vi "SyntaxToken.vi"(8 "error in":errorcluster, 9 "Error Index In":i32, 10 "Funcion Analizada":string, 11 "Parsed Expression In":T1) -> (0 "error out":errorcluster, 1 "Error Index Out":i32, 2 "Token":string[](array[string]), 3 "Parsed Expression Out":T1)   [LabVIEW 2014, in "MathLoop.lvlib"]
uses:
  MathLoop.lvlib
  TypeDefs/ParsedExpression.ctl
  TypeDefs/typeMed.ctl
  <vilib>/regexp/Match Regular Expression.xnode
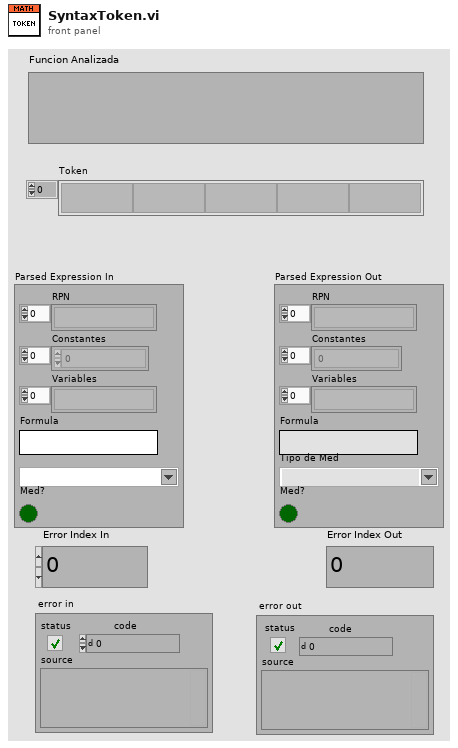
[diagram p1: front panel]
types:
  T1 = typedef "MathLoop.lvlib/ParsedExpression.ctl" = cluster{"RPN ":string[], "Constantes":sgl[], "Variables":string[], "Formula":string, "Tipo de Med":T2, "Med?":bool}
  T2 = typedef "MathLoop.lvlib/typeMed.ctl" = string
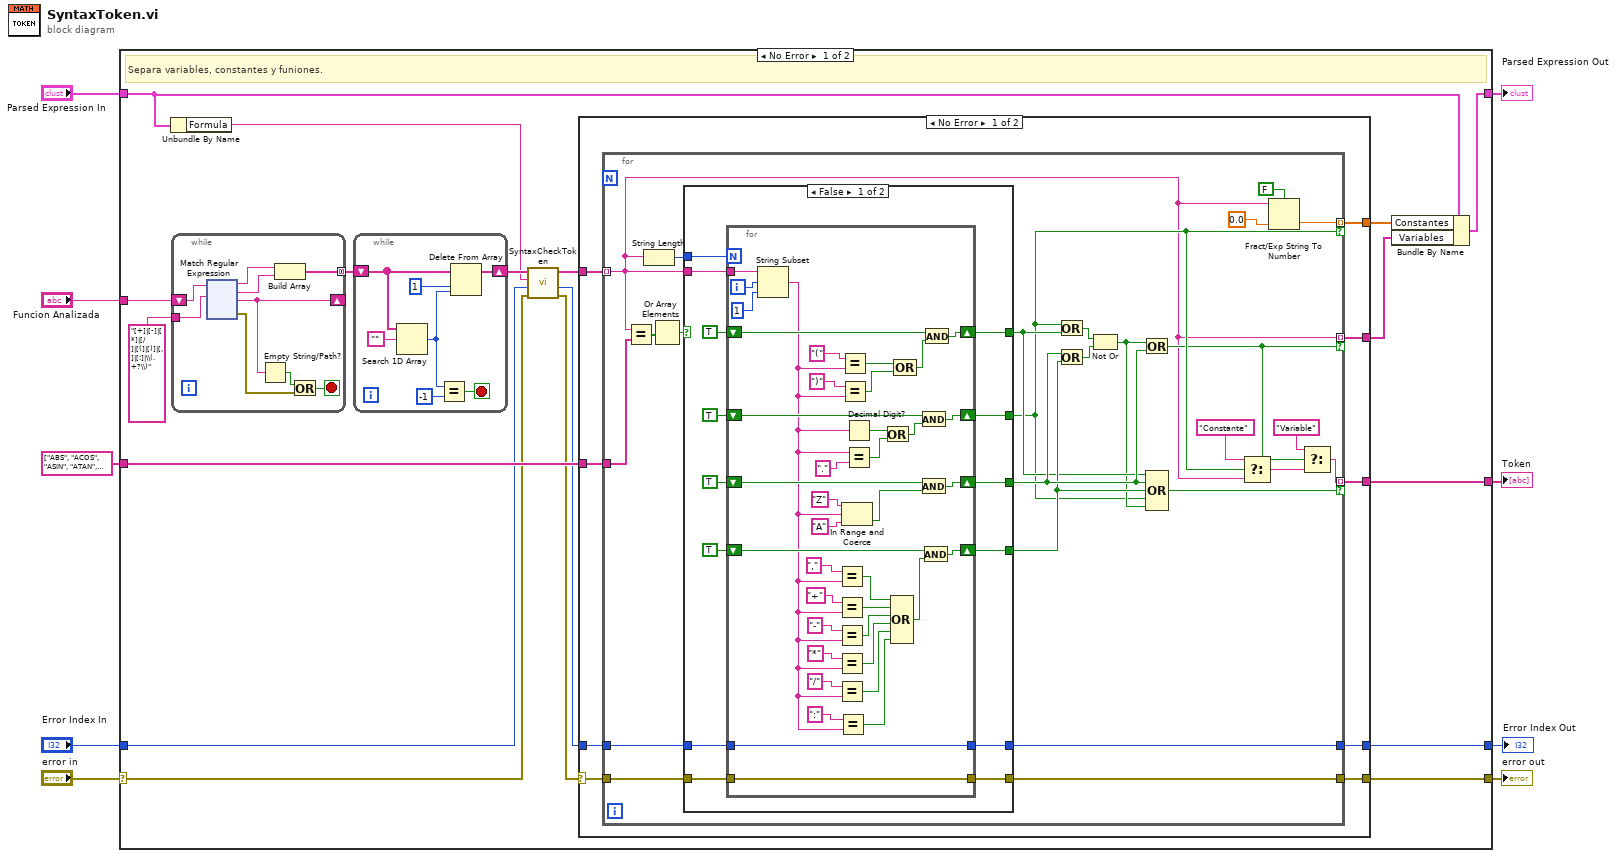
[diagram p0: block diagram]
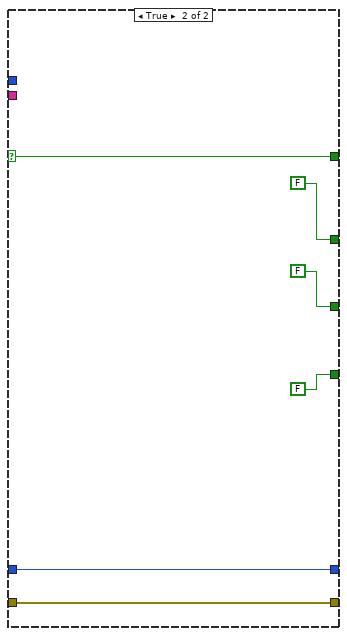
[diagram p2: hidden frame]
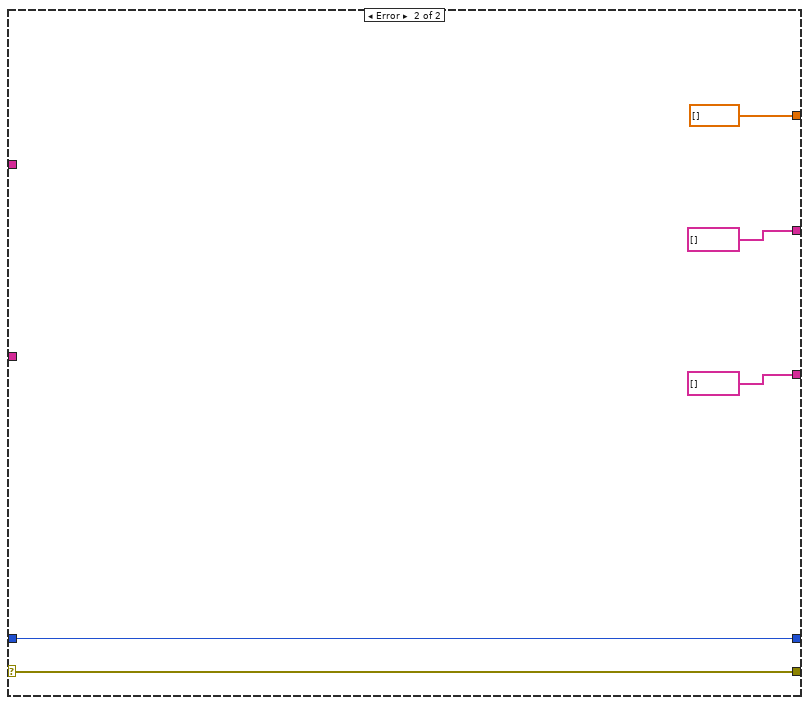
[diagram p3: hidden frame]
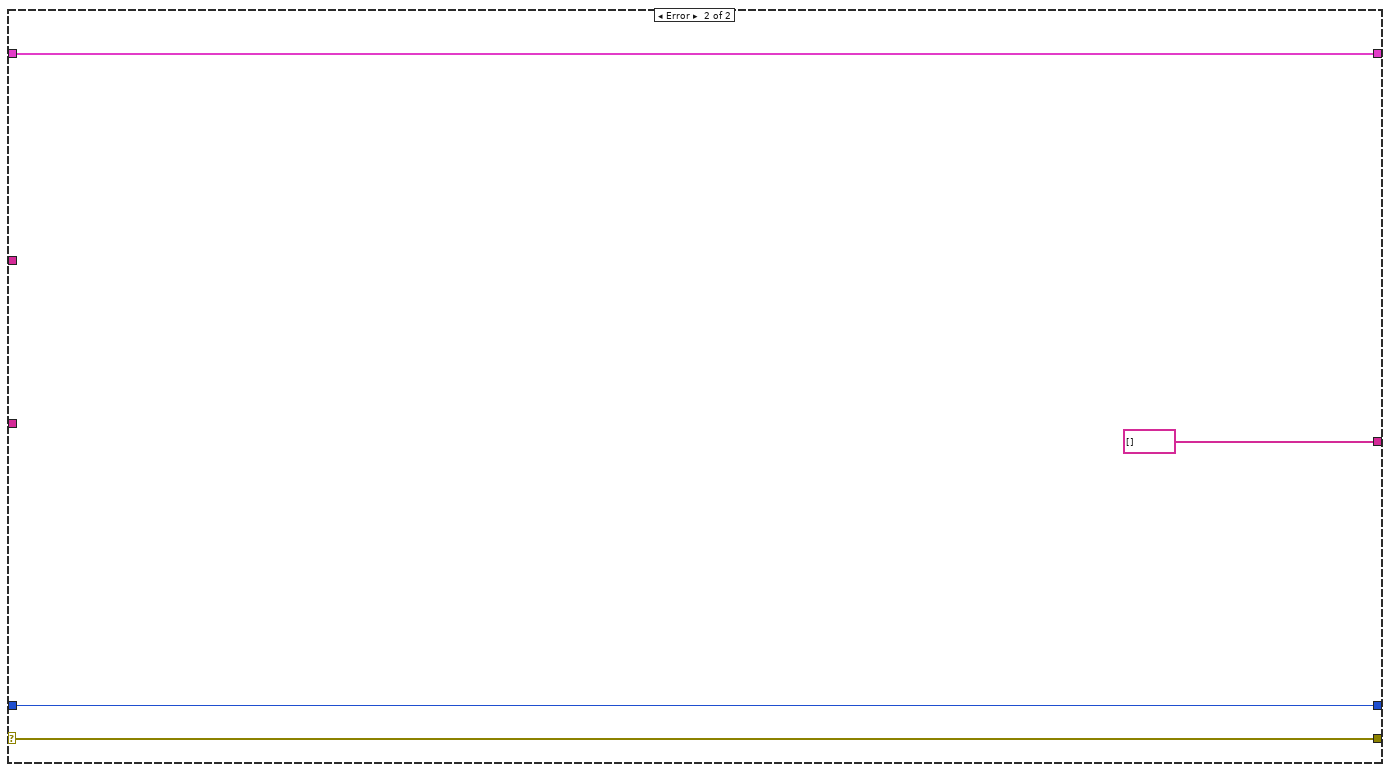
[diagram p4: hidden frame]
diagram:
  n1 = case shown="No Error" "error in" {
    selector: "error in" -> [w15 w259]
    tunnel: [w23 w259] -> w6
    tunnel: [w24 w258] -> w7
    tunnel: "Parsed Expression In" -> [w20 w258]
    tunnel: string[] ["ABS", "ACOS", "ASIN", "ATAN", "CEIL", "COS", "EXP", "FLOOR", "GETA", "GETM", "GRAD2RAD", "LOG", "MAX", "MIN", "NEG", "POW", "RAD2GRAD", "ROUND", "SIN", "SQRT", "TAN", "TRUNC"] ("Funciones") -> [w22 _]
    tunnel: [w21 string[] []] -> w4
    tunnel: "Funcion Analizada" -> [w19 _]
    tunnel: "Error Index In" -> [w13 w256]
    tunnel: [w11 w256] -> w1
    frame No Error {
      # "Separa variables, constantes y funiones."
      n2 = Unbundle By Name(w20) -> ("Formula"=w16:string)
      n3 = while {
        tunnel: "[+]|[-]|[*]|[/]|[(]|[)]|[,]|[:]|\\(.+?\\)" ("regular expression") -> [w140]
        shift-right: [w139] -> _
        shift-left: w19 -> [w141]
        tunnel: [w138] -> w26 mode=concatenating
        stop <- w134 stop-if-true
        n4 = xnode "Match Regular Expression"("input string"=w141, "regular expression"=w140) -> ("before match"=w137:string, "whole match"=w136:string, "after match"=w139:string, "error out"=w133:errorcluster)  [unwired: 4 in, 1 out]
        n5 = Empty String/Path?(string/path=w139) -> (empty?=w135:bool)
        n6 = Build Array(w137, w136) -> (w138:string[])
        n7 = Or(x=w135, y=w133) -> (x .or. y?=w134:bool)
      }
      n8 = while {
        shift-right: [w126] -> w17
        shift-left: w26 -> [w130]
        stop <- w129 stop-if-true
        n9 = Search 1D Array(1D array=w130, element="") -> (index of element=w128:i32)  [unwired: 1 in]
        n10 = Equal?(x=w128, y=-1) -> (x = y?=w129:bool)
        n11 = Delete From Array(array=w130, length=1, index=w128) -> (array with subset deleted=w126:string[])  [unwired: 1 out]
      }
      n12 = call "SyntaxCheckToken.vi"("error in"=w15, "Error Index In"=w13, "Funcion"=w16, "SyntaxChek In"=w17) -> ("error out"=w14:errorcluster, "Error Index Out"=w12:i32, "SyntaxChek Out"=w18:string[])  [unwired: 3 in]
      n13 = case shown="No Error" w14 {
        selector: w14 -> [w31 w125]
        tunnel: [w36 string[] []] -> w25
        tunnel: [w35 w125] -> w23
        tunnel: w22 -> [w34 _]
        tunnel: [w33 string[] []] -> w21
        tunnel: w18 -> [w32 _]
        tunnel: w12 -> [w30 w122]
        tunnel: [w29 w122] -> w11
        tunnel: [w28 sgl[] []] -> w10
        frame No Error {
          n14 = for {
            tunnel: w32 -> [w40] mode=indexing
            tunnel: [w48] -> w28 mode=indexing if=w46
            tunnel: [w40] -> w36 mode=indexing if=w44
            tunnel: [w41] -> w33 mode=indexing if=w58
            tunnel: w34 -> [w49]
            tunnel: w31 -> [w50]
            tunnel: [w51] -> w35
            tunnel: w30 -> [w39]
            tunnel: [w38] -> w29
            n15 = Equal?(x=w40, y=w49) -> (x = y?=w60:bool[])
            n16 = String Length(string=w40) -> (length=w61:i32)
            n17 = Or Array Elements(Boolean array=w60) -> (logical OR=w59:bool)
            n18 = case shown="False" w59 {
              selector: w59 -> [_ w120]
              tunnel: w61 -> [w75 _]
              tunnel: w40 -> [w71 _]
              tunnel: [w69 w120] -> w53
              tunnel: [w68 FALSE ("digit?")] -> w54
              tunnel: [w66 FALSE ("digit?")] -> w55
              tunnel: [w67 FALSE ("digit?")] -> w46
              tunnel: [w65 w116] -> w51
              tunnel: w50 -> [w64 w116]
              tunnel: w39 -> [w63 w115]
              tunnel: [w62 w115] -> w38
              frame False {
                n19 = for {
                  N: w75 -> [_]
                  tunnel: w71 -> [w112]
                  shift-right: [w108] -> w67
                  shift-left: TRUE ("digit?") -> [w109]
                  shift-right: [w105] -> w66
                  shift-left: TRUE ("digit?") -> [w107]
                  shift-right: [w94] -> w68
                  shift-left: TRUE ("digit?") -> [w96]
                  shift-right: [w87] -> w69
                  shift-left: TRUE ("digit?") -> [w88]
                  tunnel: [w77] -> w65
                  tunnel: w64 -> [w77]
                  tunnel: w63 -> [w76]
                  tunnel: [w76] -> w62
                  i -> [w113]
                  n20 = String Subset(string=w112, offset (0)=w113, length (rest)=1 ("length (rest)")) -> (substring=w81:string)
                  n21 = Equal?(x="," ("y"), y=w81) -> (x = y?=w85:bool)
                  n22 = Equal?(x="+" ("upper limit"), y=w81) -> (x = y?=w100:bool)
                  n23 = Equal?(x="-" ("upper limit"), y=w81) -> (x = y?=w99:bool)
                  n24 = Equal?(x="*" ("upper limit"), y=w81) -> (x = y?=w98:bool)
                  n25 = Equal?(x="/" ("upper limit"), y=w81) -> (x = y?=w97:bool)
                  n26 = Equal?(x=":" ("upper limit"), y=w81) -> (x = y?=w84:bool)
                  n27 = Equal?(x="(" ("upper limit"), y=w81) -> (x = y?=w91:bool)
                  n28 = Equal?(x=")" ("upper limit"), y=w81) -> (x = y?=w92:bool)
                  n29 = In Range and Coerce(upper limit="Z", x=w81, lower limit="A" ("upper limit")) -> (In Range?=w106:bool)  [unwired: 1 out]
                  n30 = Decimal Digit?(1:w81) -> (0:w79:bool)
                  n31 = Equal?(x=w81, y=".") -> (x = y?=w78:bool)
                  n32 = Or(x=w79, y=w78) -> (x .or. y?=w80:bool)
                  n33 = Compound Arithmetic op=OR(w85, w100, w99, w98, w97, w84) -> (w95:bool)
                  n34 = Compound Arithmetic op=OR(w91, w92) -> (w93:bool)
                  n35 = And(x=w109, y=w80) -> (x .and. y?=w108:bool)
                  n36 = And(x=w107, y=w106) -> (x .and. y?=w105:bool)
                  n37 = And(x=w96, y=w95) -> (x .and. y?=w94:bool)
                  n38 = And(x=w88, y=w93) -> (x .and. y?=w87:bool)
                }
              }
              frame True {
              }
            }
            n39 = Or(x=w46, y=w53) -> (x .or. y?=w57:bool)
            n40 = Or(x=w55, y=w54) -> (x .or. y?=w56:bool)
            n41 = Not Or(1:w56, 2:w57) -> (0:w52:bool)
            n42 = Or(x=w52, y=w55) -> (x .or. y?=w44:bool)
            n43 = Compound Arithmetic op=OR(w53, w55, w54, w46, w52) -> (w58:bool)
            n44 = Select(t="Constante" ("y"), s=w46, f=w40) -> (s? t:f=w42:string)
            n45 = Fract/Exp String To Number(use system decimal point (T)=FALSE, string=w40, default (0 dbl)=sgl 0.0 ("default (0 DBL)")) -> (number=w48:sgl)  [unwired: 1 in, 1 out]
            n46 = Select(t="Variable" ("y"), s=w44, f=w42) -> (s? t:f=w41:string)
          }
        }
        frame Error {
        }
      }
      n47 = Bundle By Name(cluster=w20, "Constantes"=w10, "Variables"=w25) -> (w24:T1)
    }
    frame Error {
    }
  }
  "Parsed Expression Out" <- w7
  "error out" <- w6
  "Token" <- w4
  "Error Index Out" <- w1
